vi "UpdateData.vi"(8 "error in (no error)":errorcluster, 10 "Select Conditions Criteria":T1, 11 "object in":refnum<class "TableLogger_CSV_Actor.lvclass">) -> (0 "error out":errorcluster, 2 "Data Clusters":variant[](array[variant]), 3 "object out":refnum<class "TableLogger_CSV_Actor.lvclass">)   [LabVIEW 2014, in "TableLogger_CSV_Actor.lvlib" / "TableLogger_CSV_Actor.lvclass"]
uses:
  TableLogger_CSV_Actor.lvclass
  TableLogger_Actor/SelectConditionCriteria.ctl
  TableLogger_SQLite_Actor/SelectConditions.ctl
  TableLogger_CSV_Actor.lvclass/TableLogger_CSV_Actor.ctl
  TableLogger_Actor/TableLogger_Actor/TableLogger_Actor.lvclass
  TableLogger_SQLite_Actor/TableLogger_SQLite_Actor/TableLogger_SQLite_Actor.lvclass
  TableLogger_Actor/TableLogger_Actor.lvlib
panel:
  # "Connector Pane"
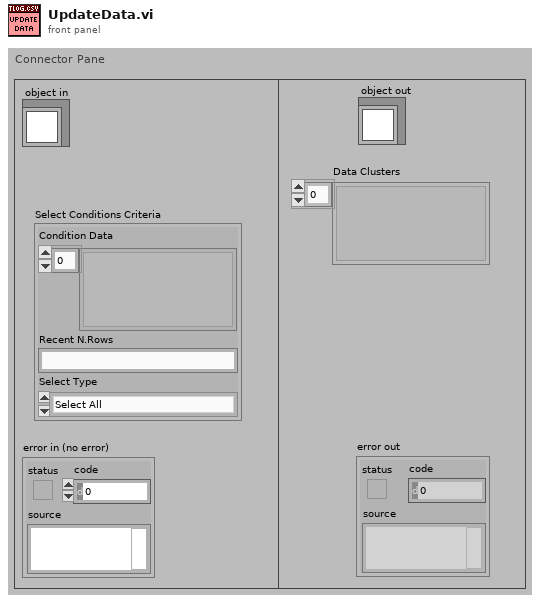
[diagram p1: front panel]
types:
  T1 = typedef "TableLogger_Actor.lvlib/SelectConditionCriteria.ctl" = cluster{"Condition Data":variant[], "Recent N.Rows":string, "Select Type":T2}
  T2 = typedef "TableLogger_Actor.lvlib/SelectConditions.ctl" = enum16{"Select All", "AND Operator", "Recent Rows", "OR Operator", "BETWEEN Operator"}
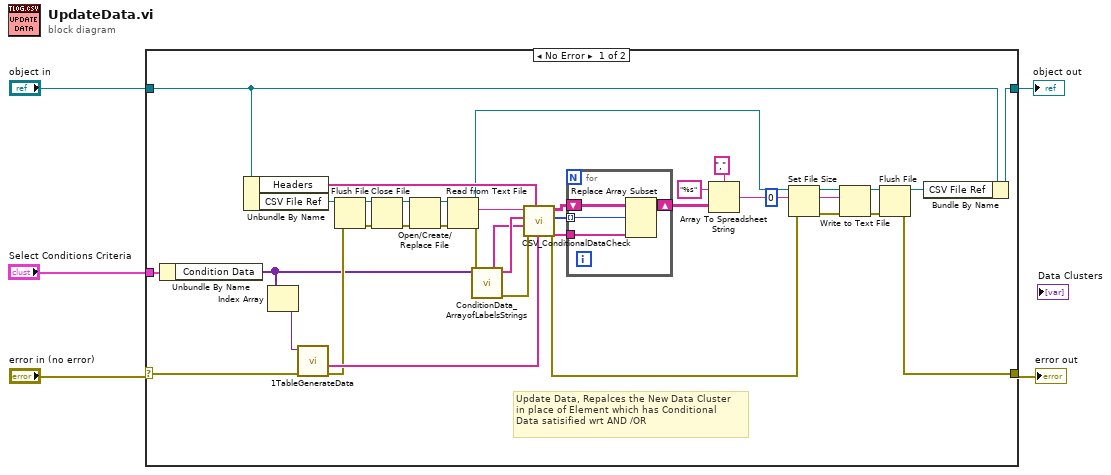
[diagram p0: block diagram]
diagram:
  n1 = case shown="No Error" "error in (no error)" {
    selector: "error in (no error)" -> [w40 w47]
    tunnel: [w32 w47] -> w5
    tunnel: [w29 w46] -> w3
    tunnel: "object in" -> [w30 w46]
    tunnel: "Select Conditions Criteria" -> [w8 _]
    frame No Error {
      # "Update Data, Repalces the New Data Cluster\nin place of Element which has Conditional \nData satisified wrt AND /OR"
      n2 = Unbundle By Name(w8) -> ("Condition Data"=w7:variant[])
      n3 = Unbundle By Name(w30) -> ("Headers"=w17:string[], "CSV File Ref"=w36:refnum<file>)
      n4 = Index Array(array=w7) -> (element=w6:variant)  [unwired: 1 in]
      n5 = call "1TableGenerateData.vi"("error in (no error)"=w40, "Cluster Variant"=w6) -> ("error out"=w35:errorcluster, "Data"=w37:string[])  [unwired: 5 in, 3 out]
      n6 = Flush File(refnum=w36, error in=w35) -> (refnum out=w22:refnum<file>, error out=w20:errorcluster)
      n7 = Close File(refnum=w22, error in=w20) -> (path=w23:path, error out=w19:errorcluster)
      n8 = Open/Create/Replace File(file path (use dialog)=w23, error in=w19) -> (refnum out=w21:refnum<file>, error out=w18:errorcluster)  [unwired: 4 in, 1 out]
      n9 = Read from Text File(file (use dialog)=w21, error in=w18) -> (refnum out=w15:refnum<file>, text=w41:string, error out=w12:errorcluster)  [unwired: 2 in, 1 out]
      n10 = call "ConditionData_ArrayofLabelsStrings.vi"("error in (no error)"=w12, "Condition Data"=w7) -> ("error out"=w11:errorcluster, "Value"=w9:string[], "Label"=w10:string[])  [unwired: 7 in]
      n11 = call "CSV_ConditionalDataCheck.vi"("Headers"=w17, "error in"=w11, "A[Data]"=w9, "A[Labels]"=w10, "Data"=w41) -> ("error out"=w24:errorcluster, "Indexes for Conditional Data"=w39:i32[], "Data in 2D"=w38:string[][])  [unwired: 2 in, 2 out]
      n12 = for {
        tunnel: w39 -> [w44] mode=indexing
        tunnel: w37 -> [w43]
        shift-right: [w42] -> w26
        shift-left: w38 -> [w45]
        n13 = Replace Array Subset(array=w45, new element=w43, index (row)=w44) -> (w42:string[][])  [unwired: 1 in]
      }
      n14 = Array To Spreadsheet String(delimiter (Tab)=",", array=w26, 3:"%s" ("format string")) -> (spreadsheet string=w25:string)
      n15 = Set File Size(4:w24, 6:i64 0 ("size (in bytes)"), 7:w15) -> (0:w16:errorcluster, 3:w14:refnum<file>)
      n16 = Write to Text File(file (use dialog)=w14, text=w25, error in=w16) -> (refnum out=w34:refnum<file>, error out=w33:errorcluster)  [unwired: 1 in, 1 out]
      n17 = Flush File(refnum=w34, error in=w33) -> (refnum out=w31:refnum<file>, error out=w32:errorcluster)
      n18 = Bundle By Name(cluster=w30, "CSV File Ref"=w31) -> (w29:refnum<class "TableLogger_CSV_Actor.lvclass">)
    }
    frame Error {
    }
  }
  "error out" <- w5
  "object out" <- w3
